vi "Teardown.vi"(8 "Error In":errorcluster, 11 "lv-libssh2 Shared Library":path=path "") -> (0 "Error Out":errorcluster)   [LabVIEW 2018, in "Tests.lvlib" / "SFTP Attributes.lvlib"]
uses:
  SFTP Attributes.lvlib
  src/Toolkit/Toolkit.lvlib
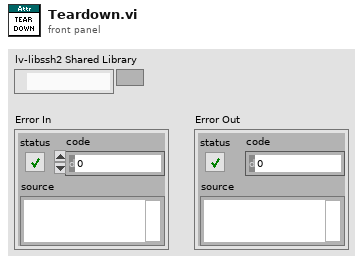
[diagram p1: front panel]
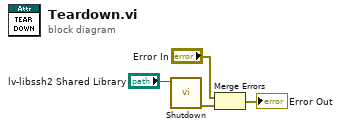
[diagram p0: block diagram]
diagram:
  n1 = call "Shutdown.vi"("lv-libssh2 Shared Library"="lv-libssh2 Shared Library") -> ("Error Out"=w4:errorcluster)  [unwired: 10 in]
  n2 = Merge Errors("Error In", w4) -> (→"Error Out":errorcluster)
